vi "tuneLeftOpenLoop_ShootDualTalonSRX.vi"(11 "F Open Loop R":dbl=0.92 format="%.5f") -> ()   [LabVIEW 2019, in "ShootDualTalonSRX_Motor_Pair.lvlib"]
uses:
  globals_ShootDualTalonSRX.vi
  ShootDualTalonSRX_Motor_Pair.lvlib
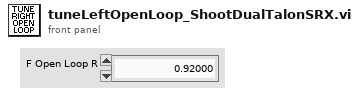
[diagram p1: front panel]
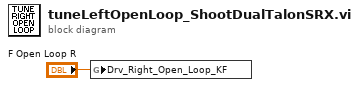
[diagram p0: block diagram]
diagram:
  n1 = global write "globals_ShootDualTalonSRX.vi" "Drv_Right_Open_Loop_KF"("F Open Loop R") -> ()
